vi "AD5781.vi"() -> ()   [LabVIEW 2014]
panel:
  out "writeIsRead":bool
  out "Readback 0 Volt":u32 format="%032b"
  out "Readback Volt":u32 format="%024b"
  in  "Set Voltage":u32 format="%024b"
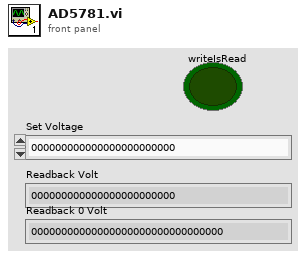
[diagram p1: front panel]
types:
  T1 = cluster{"SCLK":refnum<k21>, "CS":refnum<k21>, "MOSI":refnum<k21>, "MISO":refnum<k21>}
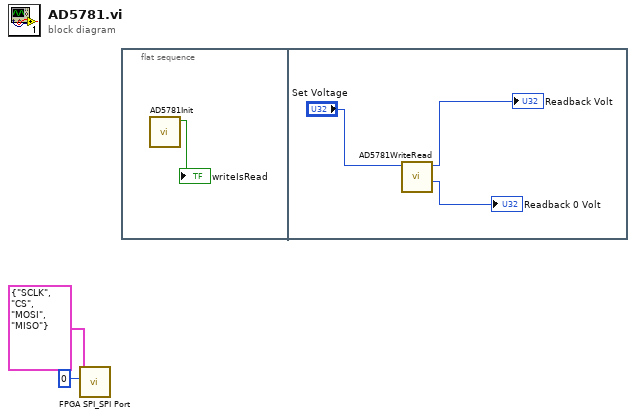
[diagram p0: block diagram]
diagram:
  n1 = call "FPGA SPI_SPI Port.vi"("Port"=i8 0, "FPGA IO"=T1 {"SCLK"="SCLK", "CS"="CS", "MOSI"="MOSI", "MISO"="MISO"}) -> ()  [unwired: 10 in]
  n2 = flat-sequence {
    frame #0 {
      n3 = call "AD5781Init.vi"() -> ("writeIsRead"=→"writeIsRead":bool)  [unwired: 11 in]
    }
    frame #1 {
      n4 = call "AD5781WriteRead.vi"("Write"="Set Voltage") -> ("Readback 0"=→"Readback 0 Volt":u32, "Readback"=→"Readback Volt":u32)  [unwired: 3 in, 3 out]
    }
  }
